vi "GetInstrParams.vi"(8 "error in (no error)":errorcluster caption="entrée d'erreur (pas d'erreur)", 10 "référence de menu":refnum<k9>, 11 "Experiment en entrée":refnum<class "Experiment.lvclass"> caption="DNL_LabVIEW Object in") -> (0 "error out":errorcluster caption="sortie d'erreur", 3 "Experiment en sortie":refnum<class "Experiment.lvclass"> caption="DNL_LabVIEW Object out")   [LabVIEW 2010, in "Experiment.lvclass"]
uses:
  Experiment.lvclass
  Experiment.lvclass/Experiment.ctl
  DevicesClass/BaseDevice/BaseDevice.lvclass
  DevicesClass/BaseDevice/Accessor/GetInstrParam.vi
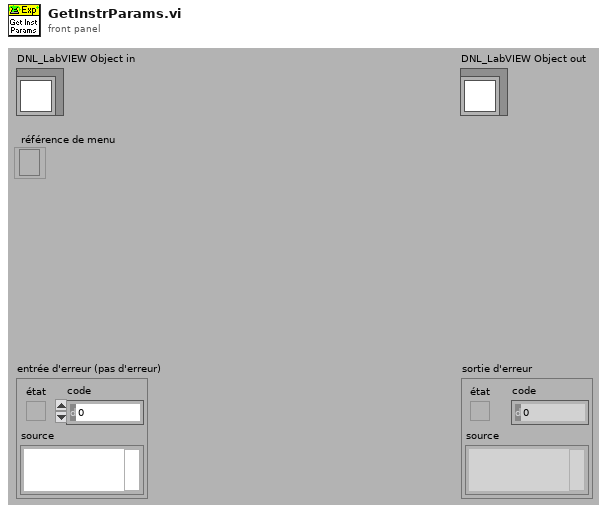
[diagram p1: front panel]
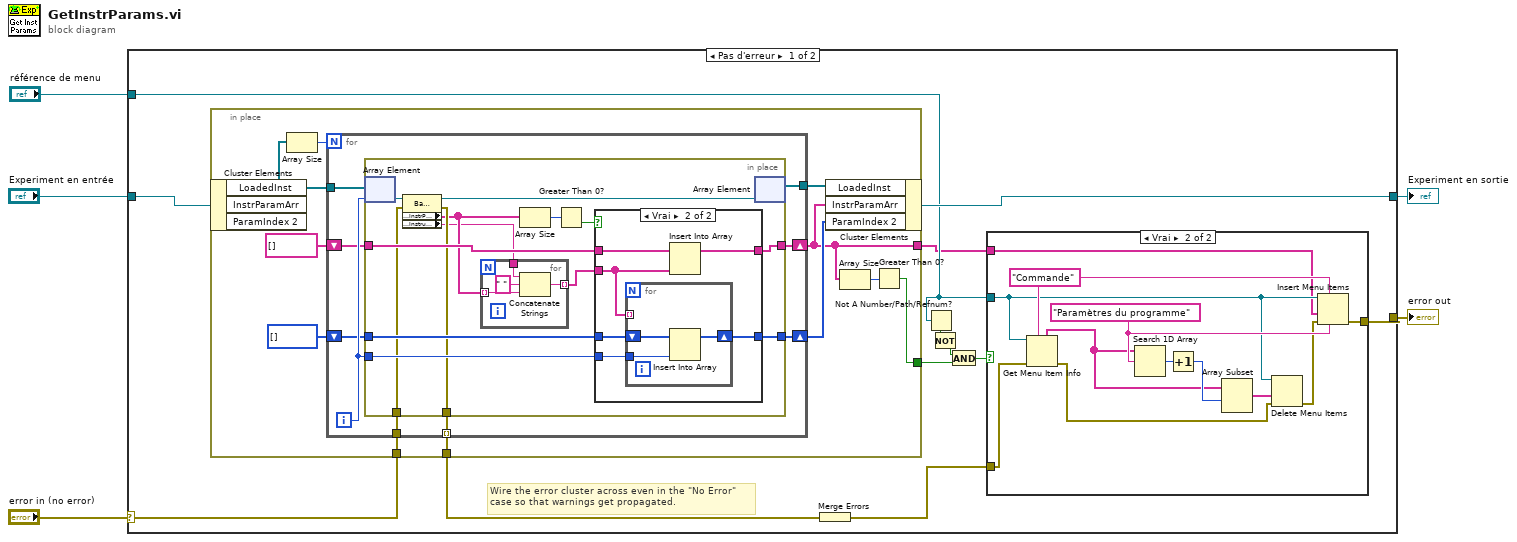
[diagram p0: block diagram]
diagram:
  n1 = case shown="Pas d'erreur" "error in (no error)" {
    selector: "error in (no error)" -> [w15 w81]
    tunnel: [w12 w81] -> w4
    tunnel: [w16 w80] -> w2
    tunnel: "Experiment en entrée" -> [w17 w80]
    tunnel: "référence de menu" -> [w8 _]
    frame No Error {
      # "Wire the error cluster across even in the \"No Error\"\ncase so that warnings get propagated."
      n2 = in-place {
        in-place-border: w15 -> [w36]
        in-place-border: [w35] -> w14
        in-place-border: [w32] -> w10
        in-place-border: [w31] -> w6
        n3 = in-place-cluster #1(w17) -> ("LoadedInst"=w37:refnum<class "BaseDevice.lvclass">[])  [unwired: 2 out]
        n4 = Array Size(array=w37) -> (size(s)=w38:i32)
        n5 = for {
          N: w38 -> [_]
          tunnel: w37 -> [w50]
          tunnel: [w49] -> w41
          shift-right: [w47] -> w34
          shift-left: i32[] [] -> [w46]
          shift-right: [w45] -> w31
          shift-left: string[] [] -> [w44]
          tunnel: w36 -> [w43]
          tunnel: [w42] -> w35 mode=indexing
          i -> [w48]
          n6 = in-place {
            in-place-border: w48 -> [w60]
            in-place-border: [w59] -> w47
            in-place-border: w46 -> [w58]
            in-place-border: [w57] -> w45
            in-place-border: w44 -> [w56]
            in-place-border: w43 -> [w55]
            in-place-border: [w54] -> w42
            n7 = in-place-array #2(w50, w48) -> (w63:refnum<class "BaseDevice.lvclass">)
            n8 = property class="BaseDevice.lvclass"(reference=w63, error in=w55) -> (reference out=w62:refnum<class "BaseDevice.lvclass">, error out=w54:errorcluster, "Accessor:InstrParam"=w53:string[], "Accessor:InstrumentName"=w52:string)
            n9 = for {
              tunnel: w53 -> [w68] mode=indexing
              tunnel: w52 -> [w66]
              tunnel: [w65] -> w51 mode=indexing
              n10 = Concatenate Strings(w66, " " ("chaîne"), w68) -> (w65:string)
            }
            n11 = Array Size(array=w53) -> (size(s)=w64:i32)
            n12 = Greater Than 0?(x=w64) -> (x > 0?=w61:bool)
            n13 = case shown="Vrai" w61 {
              tunnel: w60 -> [_ w75]
              tunnel: [w70 w76] -> w59
              tunnel: w58 -> [w70 w71]
              tunnel: w51 -> [_ w72]
              tunnel: [w69 w74] -> w57
              tunnel: w56 -> [w69 w73]
              frame False {
              }
              frame True {
                n14 = for {
                  tunnel: w75 -> [w78]
                  tunnel: w72 -> [_] mode=indexing
                  shift-right: [w79] -> w76
                  shift-left: w71 -> [w77]
                  n15 = Insert Into Array(array=w77, new element=w78) -> (w79:i32[])  [unwired: 1 in]
                }
                n16 = Insert Into Array(array=w73, new element=w72) -> (w74:string[])  [unwired: 1 in]
              }
            }
            n17 = in-place-array #2(w62) -> (w49:refnum<class "BaseDevice.lvclass">[])  [unwired: 1 out]
          }
        }
        n18 = in-place-cluster #1("LoadedInst"=w41, "InstrParamArr"=w31, "ParamIndex 2"=w34) -> (w16:refnum<class "Experiment.lvclass">)
        n19 = Array Size(array=w31) -> (size(s)=w33:i32)
        n20 = Greater Than 0?(x=w33) -> (x > 0?=w32:bool)
      }
      n21 = Merge Errors(w14) -> (w13:errorcluster)
      n22 = Not A Number/Path/Refnum?(number/path/refnum=w8) -> (NaN/Path/Refnum?=w9:bool)
      n23 = Not(x=w9) -> (.not. x?=w7:bool)
      n24 = And(x=w7, y=w10) -> (x .and. y?=w11:bool)
      n25 = case shown="Vrai" w11 {
        tunnel: w8 -> [_ w20]
        tunnel: w13 -> [w18 w22]
        tunnel: [w18 w21] -> w12
        tunnel: w6 -> [_ w19]
        frame False {
        }
        frame True {
          w29 = "Paramètres du programme" ("élément suivant")
          w25 = "Commande" ("tag de menu")
          n26 = Get Menu Item Info(7:w25, 8:w22, 11:w20) -> (0:w24:errorcluster, 5:w26:string[])  [unwired: 5 out]
          n27 = Search 1D Array(1D array=w26, element=w29) -> (index of element=w27:i32)  [unwired: 1 in]
          n28 = Increment(x=w27) -> (x+1=w30:i32)
          n29 = Array Subset(array=w26, index=w30) -> (w28:string[])  [unwired: 1 in]
          n30 = Delete Menu Items(6:w24, 7:w28, 9:w20) -> (0:w23:errorcluster)  [unwired: 1 in, 1 out]
          n31 = Insert Menu Items(4:w29, 5:w25, 6:w23, 7:w19, 9:w20) -> (0:w21:errorcluster)  [unwired: 1 in, 2 out]
        }
      }
    }
    frame Error {
    }
  }
  "error out" <- w4
  "Experiment en sortie" <- w2
